vi "Get Type Specializations.vi"(8 "error in":errorcluster) -> (0 "error out":errorcluster, 2 "type specializations":T1[](array[typedef]))   [LabVIEW 2021, in "Tree.lvlib"]
uses:
  Tree.lvlib
  <vilib>/MeasurementLink/MeasurementLink Measurement Server/Helpers/TypeDefs/Parameter Type Specialization.ctl
  <vilib>/MeasurementLink/MeasurementLink Measurement Server/Helpers/TypeDefs/Type Specialization.ctl
  <vilib>/MeasurementLink/MeasurementLink Measurement Server/Helpers/TypeDefs/Type Specialization Key.ctl
  <vilib>/MeasurementLink/MeasurementLink Measurement Server/MeasurementLink Measurement Server.lvlib
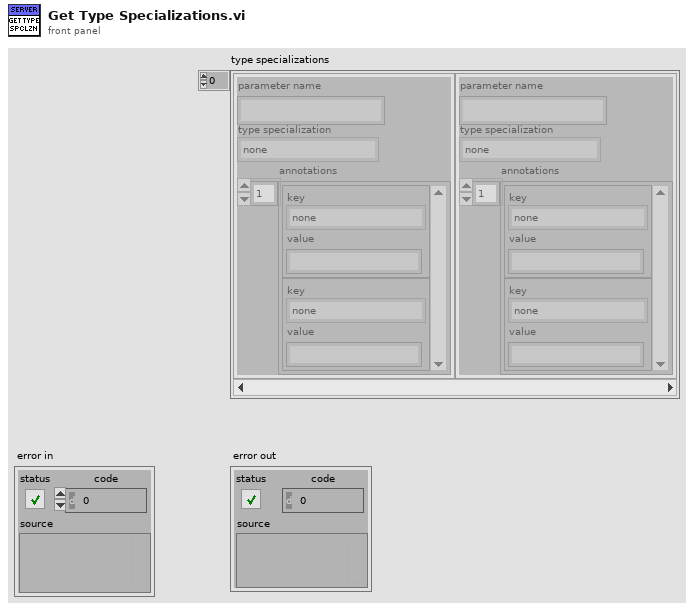
[diagram p1: front panel]
types:
  T1 = typedef "MeasurementLink Measurement Server.lvlib/Parameter Type Specialization.ctl" = cluster{"parameter name":string, "type specialization":T2, "annotations":cluster{"key":T3, "value":string}[]}
  T2 = typedef "MeasurementLink Measurement Server.lvlib/Type Specialization.ctl" = enum16{"none", "pin", "path", "enum"}
  T3 = typedef "MeasurementLink Measurement Server.lvlib/Type Specialization Key.ctl" = enum16{"none", "pin.instrument_type", "enum.values"}
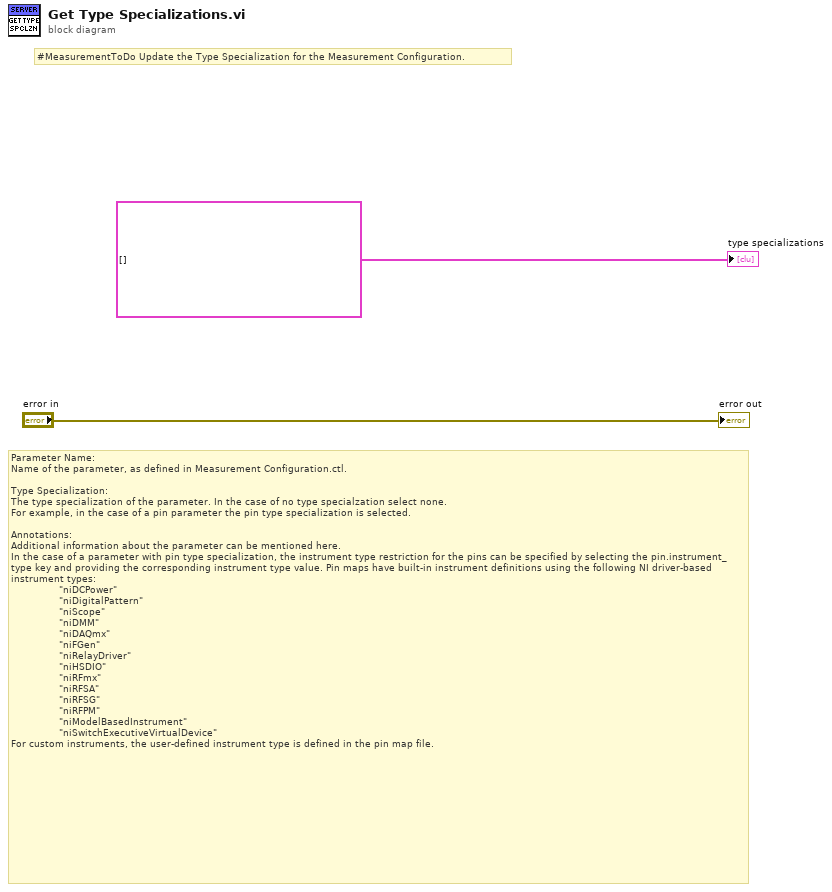
[diagram p0: block diagram]
diagram:
  # "Parameter Name: \nName of the parameter, as defined in Measurement Configuration.ctl.\n\nType Specialization: \nThe type specialization of the parameter. In the case of no type specialzation select none. \nFor example, in the case of a pin parameter the pin type specialization is selected.\n\nAnnotations:\nAdditional information about the parameter can be mentioned here.\nIn the case of a parameter with pin type specialization, the instrument type restriction for the pins can be specified by selecting the pin.instrument_type key and providing the corresponding instrument type value. Pin maps have built-in instrument definitions using the following NI driver-based instrument types:\n                \"niDCPower\"\n                \"niDigitalPattern\"\n                \"niScope\"\n                \"niDMM\"\n                \"niDAQmx\"\n                \"niFGen\"\n                \"niRelayDriver\"\n                \"niHSDIO\"\n                \"niRFmx\"\n                \"niRFSA\"\n                \"niRFSG\"\n                \"niRFPM\"\n                \"niModelBasedInstrument\"\n                \"niSwitchExecutiveVirtualDevice\"\nFor custom instruments, the user-defined instrument type is defined in the pin map file."
  # "#MeasurementToDo Update the Type Specialization for the Measurement Configuration."
  "type specializations" <- T1[] []
  "error out" <- "error in"
